vi "http write header.vi"(8 "error in (no error)":errorcluster, 10 "application request":T1, 11 "TCP Network Connection in":refnum<k5>) -> (0 "error out":errorcluster, 3 "TCP Network Connection out":refnum<k5>)   [LabVIEW 2016, in "Basic HTTP server.lvclass"]
uses:
  Basic HTTP server.lvclass
  http response.ctl
  http response packet type.ctl
  HTTP headers/http header data.ctl
  HTTP headers/http headers.lvlib
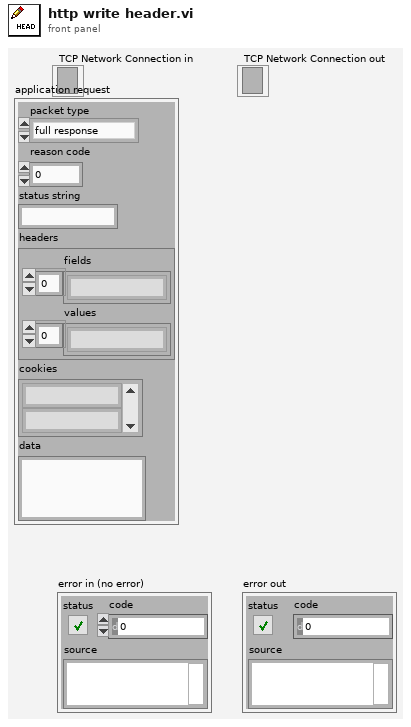
[diagram p1: front panel]
types:
  T1 = typedef "Basic HTTP server.lvclass/http response.ctl" = cluster{"packet type":T2, "reason code":u16, "status string":string, "headers":T3, "cookies":string[], "data":string}
  T2 = typedef "Basic HTTP server.lvclass/http response packet type.ctl" = enum16{"full response", "header only", "data only", "last data"}
  T3 = typedef "http headers.lvlib/http header data.ctl" = cluster{"fields":string[], "values":string[]}
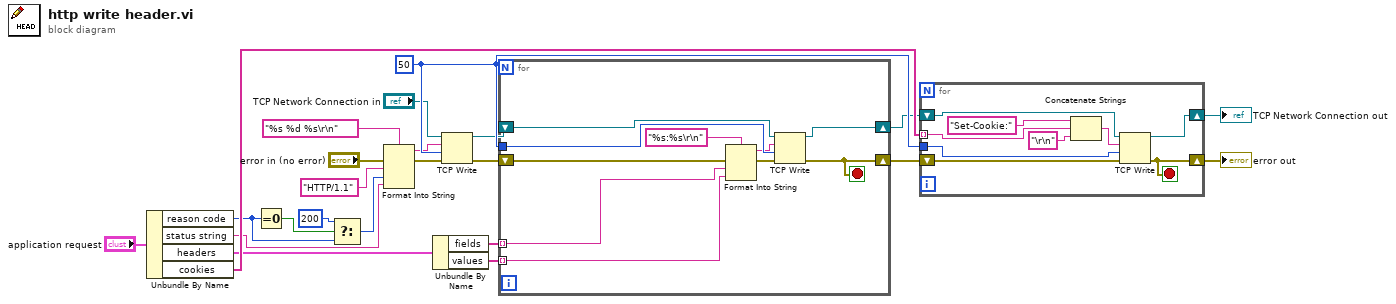
[diagram p0: block diagram]
diagram:
  w22 = 50 ("timeout ms (25000)")
  n1 = Unbundle By Name("application request") -> ("reason code"=w5:u16, "status string"=w10:string, "headers"=w3:T3, "cookies"=w19:string[])
  n2 = Equal To 0?(x=w5) -> (x = 0?=w7:bool)
  n3 = Select(t=u16 200, s=w7, f=w5) -> (s? t:f=w4:u16)
  n4 = Format Into String(format string="%s %d %s\r\n", error in="error in (no error)", "HTTP/1.1" ("input 1"), w4, w10) -> (resulting string=w13:string, error out=w14:errorcluster)  [unwired: 1 in]
  n5 = Unbundle By Name(w3) -> ("fields"=w2:string[], "values"=w1:string[])
  n6 = TCP Write(connection ID="TCP Network Connection in", data in=w13, error in (no error)=w14, 9:w22) -> (connection ID out=w15:refnum<k5>, error out=w16:errorcluster)  [unwired: 1 out]
  n7 = for {
    shift-right: [w33] -> w17
    shift-left: w15 -> [w31]
    shift-right: [w28] -> w18
    shift-left: w16 -> [w30]
    tunnel: w22 -> [w32]
    tunnel: w2 -> [w29] mode=indexing
    tunnel: w1 -> [w27] mode=indexing
    stop <- w28 stop-if-true
    n8 = Format Into String(format string="%s:%s\r\n", error in=w30, w29, w27) -> (resulting string=w24:string, error out=w26:errorcluster)  [unwired: 1 in]
    n9 = TCP Write(connection ID=w31, data in=w24, error in (no error)=w26, 9:w32) -> (connection ID out=w33:refnum<k5>, error out=w28:errorcluster)  [unwired: 1 out]
  }
  n10 = for {
    shift-right: [w42] -> w20
    shift-left: w17 -> [w41]
    shift-right: [w39] -> w21
    shift-left: w18 -> [w40]
    tunnel: w19 -> [w36] mode=indexing
    tunnel: w22 -> [w34]
    stop <- w39 stop-if-true
    n11 = Concatenate Strings("Set-Cookie:" ("string"), w36, "\r\n" ("format string")) -> (w35:string)
    n12 = TCP Write(connection ID=w41, data in=w35, error in (no error)=w40, 9:w34) -> (connection ID out=w42:refnum<k5>, error out=w39:errorcluster)  [unwired: 1 out]
  }
  "error out" <- w21
  "TCP Network Connection out" <- w20
